vi "start.vi"(8 "error in (no error)":errorcluster, 11 "DL090211ImageAssemblerScaffold in":refnum<class "ImageAssemblerDL090211Scaffold.lvclass">) -> (0 "error out":errorcluster, 3 "DL090211ImageAssemblerScaffold out":refnum<class "ImageAssemblerDL090211Scaffold.lvclass">)   [LabVIEW 2010, in "ImageAssemblerDL090211Scaffold.lvclass"]
uses:
  ImageAssemblerDL090211Scaffold.lvclass
  GenericImageAssembler/GenericImageAssembler/GenericImageAssembler.lvclass
  common/classes/Image/Image/Image.lvclass
  ImageAssemblerDL090211Scaffold.lvclass/ImageAssemblerDL090211Scaffold.ctl
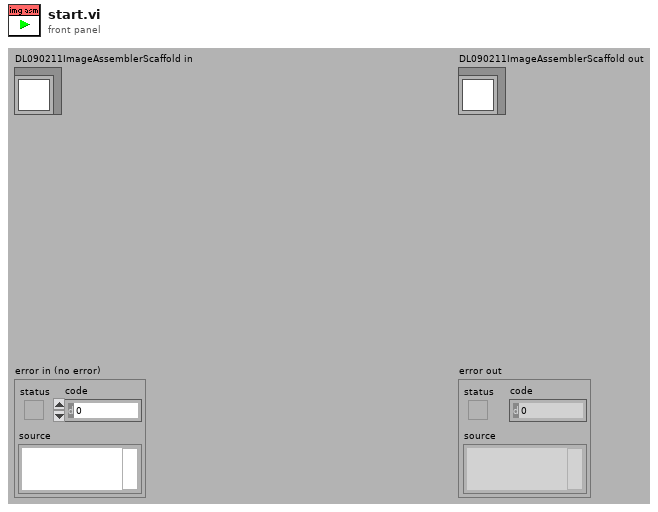
[diagram p1: front panel]
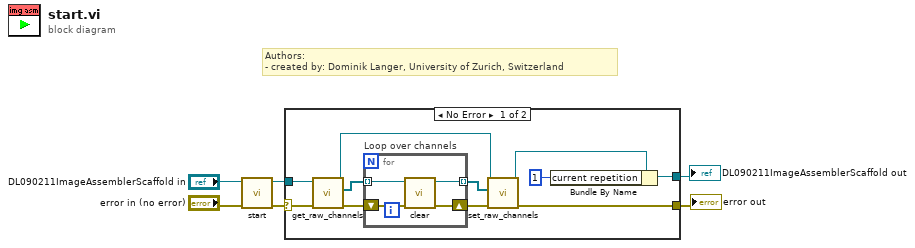
[diagram p0: block diagram]
diagram:
  # "Authors: \n- created by: Dominik Langer, University of Zurich, Switzerland"
  n1 = call-parent "start.vi"("error in (no error)"="error in (no error)", "GenericToplevelComponent in"="DL090211ImageAssemblerScaffold in") -> ("error out"=w5:errorcluster, "GenericToplevelComponent out"=w3:refnum<class "ImageAssemblerDL090211Scaffold.lvclass">)  [unwired: 8 in]
  n2 = case shown="No Error" w5 {
    selector: w5 -> [w7 w23]
    tunnel: [w15 w23] -> w1
    tunnel: [w10 w22] -> w2
    tunnel: w3 -> [w8 w22]
    frame No Error {
      n3 = call-dynamic "get_raw_channels.vi"("error in (no error)"=w7, "DL090211ImageAssemblerScaffold.lvclass in"=w8) -> ("error out"=w17:errorcluster, "raw channels"=w14:refnum<class "Image.lvclass">[], "DL090211ImageAssemblerScaffold.lvclass out"=w12:refnum<class "ImageAssemblerDL090211Scaffold.lvclass">)  [unwired: 7 out]
      n4 = for "Loop over channels" {
        tunnel: w14 -> [w19] mode=indexing
        tunnel: [w18] -> w13 mode=indexing
        shift-right: [w20] -> w16
        shift-left: w17 -> [w21]
        n5 = call-dynamic "clear.vi"("error in (no error)"=w21, "Image in"=w19) -> ("error out"=w20:errorcluster, "Image out"=w18:refnum<class "Image.lvclass">)  [unwired: 8 out]
      }
      n6 = call "set_raw_channels.vi"("error in (no error)"=w16, "raw channels"=w13, "DL090211ImageAssemblerScaffold.lvclass in"=w12) -> ("error out"=w15:errorcluster, "DL090211ImageAssemblerScaffold.lvclass out"=w11:refnum<class "ImageAssemblerDL090211Scaffold.lvclass">)  [unwired: 7 out]
      n7 = Bundle By Name(cluster=w11, "current repetition"=1) -> (w10:refnum<class "ImageAssemblerDL090211Scaffold.lvclass">)
    }
    frame Error {
    }
  }
  "error out" <- w1
  "DL090211ImageAssemblerScaffold out" <- w2
